vi "Accessor - Get.vi"(8 "error in (no error)":errorcluster, 9 "default values":variant[](array[variant]), 10 "keys":string[](array[string]), 11 "uData in":refnum<class "uData.lvclass">) -> (0 "error out":errorcluster, 1 "values":variant[](array[variant]), 3 "uData out":refnum<class "uData.lvclass">, 4 "found?":bool[](array[boolean]))   [LabVIEW 2023, in "uLib.lvlib" / "uData.lvclass"]
doc: "This is a (GET) accessor to use by all other methods. It performs key conditioning, array size match check and calls the dynamic dispatch inline operation. It handles output values on error as well."
uses:
  uData.lvclass
  uData.lvclass/uData.ctl
  Condition Tag Name.vi
  Blank Key Reserved String.vi
  <vilib>/Utility/error.llb/Error Cluster From Error Code.vi
  <vilib>/ErrorRing/Error Ring.xnode
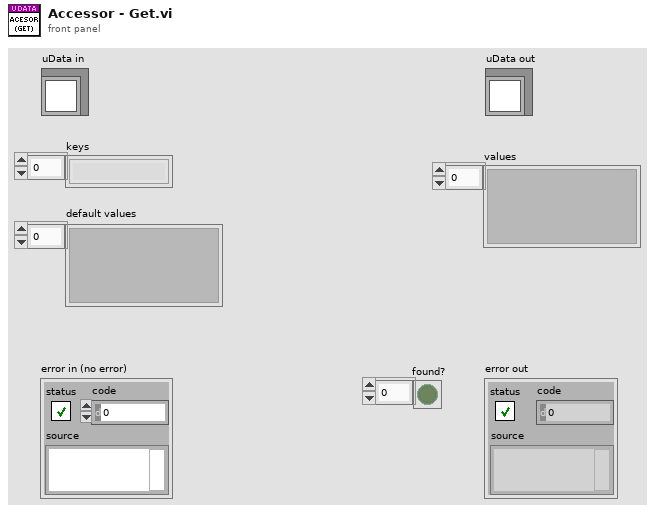
[diagram p1: front panel]
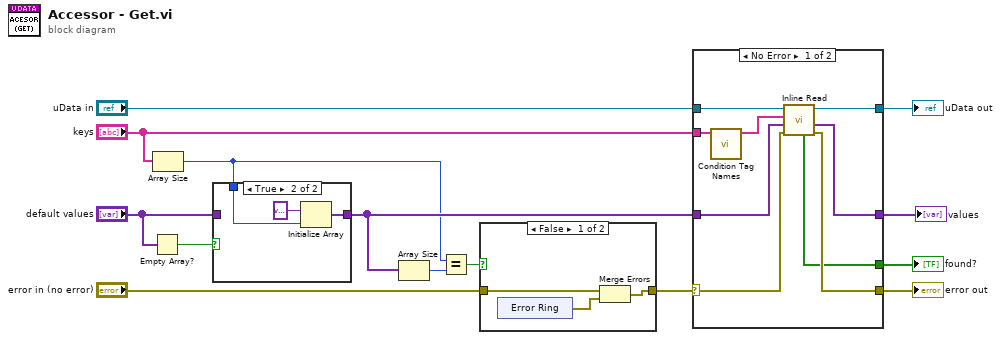
[diagram p0: block diagram]
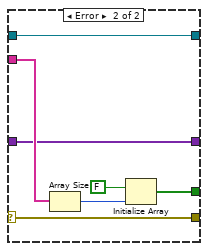
[diagram p3: hidden frame]
diagram:
  n1 = Empty Array?(array="default values") -> (empty?=w4:bool)
  n2 = Array Size(array="keys") -> (size(s)=w1:i32)
  n3 = case shown="True" w4 {
    tunnel: "default values" -> [w15 _]
    tunnel: [w15 w18] -> w2
    tunnel: w1 -> [_ w16]
    frame False {
    }
    frame True {
      n4 = Initialize Array(variant, w16) -> (w18:variant[])
    }
  }
  n5 = Array Size(array=w2) -> (size(s)=w9:i32)
  n6 = Equal?(x=w1, y=w9) -> (x = y?=w8:bool)
  n7 = case shown="False" w8 {
    tunnel: "error in (no error)" -> [w20 w27]
    tunnel: [w21 w27] -> w6
    frame False {
      n8 = xnode "Error Ring"() -> ("error out"=w19:errorcluster)
      n9 = Merge Errors(w20, w19) -> (w21:errorcluster)
    }
    frame True {
    }
  }
  n10 = case shown="No Error" w6 {
    selector: w6 -> [w34 w43]
    tunnel: [w33 w43] -> w14
    tunnel: [w36 w42] -> w12
    tunnel: "uData in" -> [w35 w42]
    tunnel: [w32 w38] -> w11
    tunnel: w2 -> [w31 w37]
    tunnel: "keys" -> [w30 w39]
    tunnel: [w29 w37] -> w5
    frame No Error {
      n11 = call "Condition Tag Names.vi"("tags in"=w30) -> ("tags out"=w28:string[])  [unwired: 10 in]
      n12 = call "Inline Read.vi"("error in (no error)"=w34, "default values"=w31, "keys"=w28, "uData in"=w35) -> ("error out"=w33:errorcluster, "values"=w29:variant[], "uData out"=w36:refnum<class "uData.lvclass">, "found?"=w32:bool[])  [unwired: 4 in]
    }
    frame Error {
      n13 = Array Size(array=w39) -> (size(s)=w41:i32)
      n14 = Initialize Array(FALSE, w41) -> (w38:bool[])
    }
  }
  "error out" <- w14
  "uData out" <- w12
  "found?" <- w11
  "values" <- w5
